vi "Write Signal Refnum.vi"(8 "error in (no error)":errorcluster, 10 "Signal Refnum":refnum<vi>, 11 "Configuration UI in":refnum<class "Configuration UI.lvclass">) -> (0 "error out":errorcluster, 3 "Configuration UI out":refnum<class "Configuration UI.lvclass">)   [LabVIEW 2023, in "Configuration UI.lvlib" / "Configuration UI.lvclass"]
uses:
  Project/Configuration UI.lvclass
  Project/Configuration UI.lvclass/Configuration UI.ctl
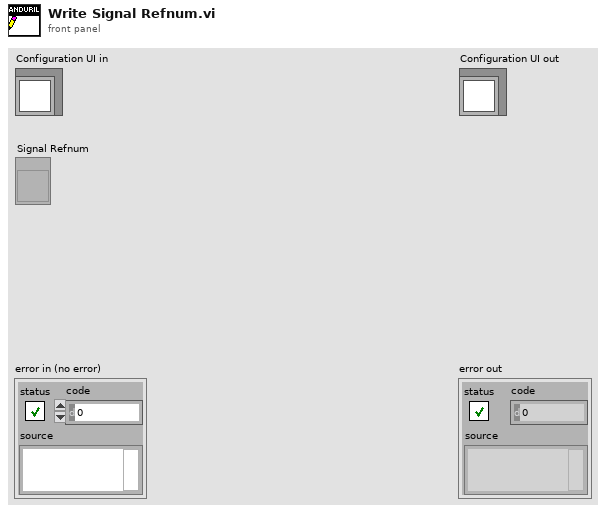
[diagram p1: front panel]
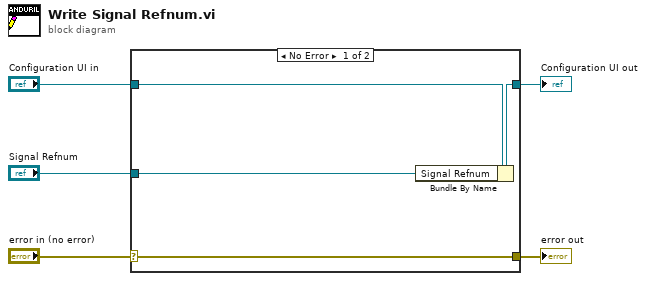
[diagram p0: block diagram]
diagram:
  n1 = case shown="No Error" "error in (no error)" {
    selector: "error in (no error)" -> [w9 w10]
    tunnel: [w9 w10] -> w4
    tunnel: [w7 w11] -> w2
    tunnel: "Configuration UI in" -> [w8 w11]
    tunnel: "Signal Refnum" -> [w6 _]
    frame No Error {
      n2 = Bundle By Name(cluster=w8, "Signal Refnum"=w6) -> (w7:refnum<class "Configuration UI.lvclass">)
    }
    frame Error {
    }
  }
  "error out" <- w4
  "Configuration UI out" <- w2
